vi "Close.vi"(8 "error in (no error)":errorcluster, 11 "TCP Client in":refnum<class "TCP Client.lvclass">) -> (0 "error out":errorcluster, 3 "TCP Client out":refnum<class "TCP Client.lvclass">)   [LabVIEW 2012, in "Stream-TCP.lvlib" / "TCP Client.lvclass"]
uses:
  TCP Client.lvclass
  Client Command.ctl
  Stream-TCP.lvlib
  Connection State.ctl
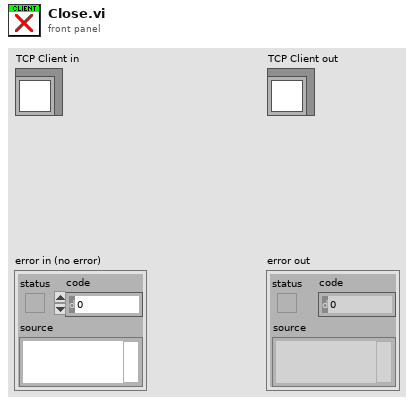
[diagram p1: front panel]
types:
  T1 = typedef "Stream-TCP.lvlib/TCP Client.lvclass/Connection State.ctl" = enum16{"Closed", "Idle", "Connecting", "Connected", "Shutdown"}
  T2 = typedef "Stream-TCP.lvlib/Client Command.ctl" = enum16{"Connect", "Close", "Shutdown", "Reconnect"}
  T3 = typedef "Stream-TCP.lvlib/Client Command Queue.ctl" = refnum<queue>
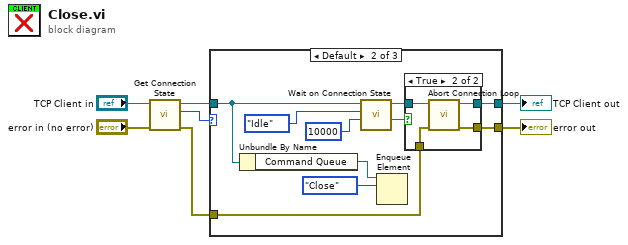
[diagram p0: block diagram]
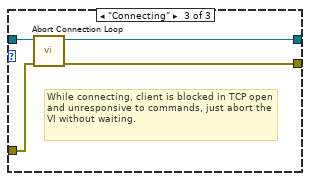
[diagram p4: hidden frame]
diagram:
  n1 = call "Get Connection State.vi"("error in (no error)"="error in (no error)", "TCP Client in"="TCP Client in") -> ("error out"=w2:errorcluster, "State"=w4:T1, "TCP Client out"=w5:refnum<class "TCP Client.lvclass">)  [unwired: 7 in]
  n2 = case shown="Default" w4 {
    tunnel: [w9 w13 w27] -> w7
    tunnel: w2 -> [w8 w12 w28]
    tunnel: [w8 w11 w26] -> w3
    tunnel: w5 -> [w9 w10 w29]
    frame "Closed", "Idle" {
    }
    frame Default {
      n3 = Unbundle By Name(w10) -> ("Command Queue"=w19:T3)
      n4 = call "Wait on Connection State.vi"("Timeout ms (-1)"=10000, "Connection State"=Connection_State."Idle", "TCP Client in"=w10) -> ("Timed Out?"=w15:bool, "TCP Client out"=w14:refnum<class "TCP Client.lvclass">)  [unwired: 6 in, 1 out]
      n5 = Enqueue Element(queue=w19, element=Client_Command."Close") -> ()  [unwired: 2 in, 3 out]
      n6 = case shown="True" w15 {
        tunnel: w14 -> [w21 w25]
        tunnel: [w21 w24] -> w13
        tunnel: w12 -> [w20 w23]
        tunnel: [w20 w22] -> w11
        frame False {
        }
        frame True {
          n7 = call "Abort Connection Loop.vi"("error in (no error)"=w23, "TCP Client in"=w25) -> ("error out"=w22:errorcluster, "TCP Client out"=w24:refnum<class "TCP Client.lvclass">)  [unwired: 8 in]
        }
      }
    }
    frame "Connecting" {
      # "While connecting, client is blocked in TCP open and unresponsive to commands, just abort the VI without waiting."
      n8 = call "Abort Connection Loop.vi"("error in (no error)"=w28, "TCP Client in"=w29) -> ("error out"=w26:errorcluster, "TCP Client out"=w27:refnum<class "TCP Client.lvclass">)  [unwired: 8 in]
    }
  }
  "error out" <- w3
  "TCP Client out" <- w7
